vi "Thread 1.vi"(8 "error in (no error)":errorcluster, 11 "MyApp in":refnum<class "MyApp.lvclass">) -> (0 "error out":errorcluster, 3 "MyApp out":refnum<class "MyApp.lvclass">)   [LabVIEW 2012, in "MyApp.lvlib" / "MyApp.lvclass"]
uses:
  MyApp.lvclass
  HGF_LVC/HGF_BaseClasses/HGF_Event/HGF_Event.lvclass
  HGF_LVC/HGF_BaseClasses/HGF_Stop/HGF_Stop.lvclass
  HGF_LVC/HGF_BaseClasses/HGF_VariantDataObject/HGF_VariantDataObject.lvclass
  HGF_DataAnalyzer/WfmAnalysator/WfmAnalysator.lvclass
  HGF_DataAnalyzer/Wfm_Amplitude/Wfm_Amplitude.lvclass
  HGF_DataAnalyzer/Wfm_PulseMeasurement/Wfm_PulseMeasurement.lvclass
  MyApp.lvclass/MyApp.ctl
  HGF_DataAnalyzer/HGF_DataAnalysis/HGF_DataAnalysis.lvclass
  <vilib>/Utility/error.llb/DialogType.ctl
  <vilib>/measure/mascope.llb/Pulse Measurements 1 chan.vi
  <vilib>/measure/mascope.llb/Amplitude and Levels 1 chan.vi
  HGF_LVC/HGF_ApplicationBaseClasses/HGF_Application/HGF_Application.lvclass
  <vilib>/measure/NI_MABase.lvlib
  <vilib>/measure/NI_MAPro.lvlib
  HGF_LVC/HGF_BaseClasses/HGF_Composite/HGF_Composite.lvclass
panel:
  out "amplitude 3":dbl
  out "period 2":dbl format="%.2g"
  out "measurement info":T1
  out "Waveform Graph":waveform(dbl)(graph)
  out "low state level":dbl
  out "high state level":dbl
  out "amplitude 2":dbl format="%.2p"
  out "duty cycle":dbl
  out "pulse duration":dbl
  out "period":dbl format="%.2g"
  out "Analysis Error":errorcluster
  in  "sampling info":cluster{"Fs":dbl, "#s":dbl}={"Fs"=1000.0, "#s"=1000.0} {"Fs" format="%.2p"}
  in  "square wave duty cycle (%)":dbl=50.0 format="%0.2f"
  in  "amplitude":dbl=1.0 format="%0.2p"
  in  "frequency":dbl=10.0 format="%0.2p"
  in  "offset":dbl format="%0.2p"
  in  "signal type":T2(ring)
  in  "Generate Waveform":bool
  out "Iteration":i32
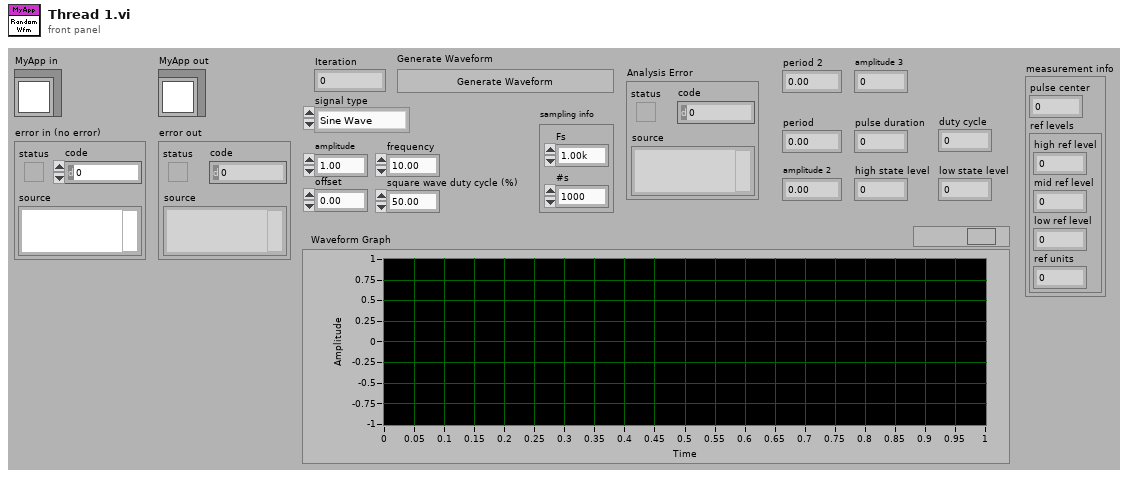
[diagram p1: front panel]
types:
  T1 = cluster{"pulse center":dbl, "ref levels":cluster{"high ref level":dbl, "mid ref level":dbl, "low ref level":dbl, "ref units":u16}}
  T2 = enum16{"Sine Wave", "Triangle Wave", "Square Wave", "Sawtooth Wave"}
  T3 = cluster{"seconds since 1Jan1904":timestamp, "message":string}
  T4 = typedef "DialogType.ctl" = u16
  T5 = cluster{"seconds since 1Jan1904":timestamp, string}
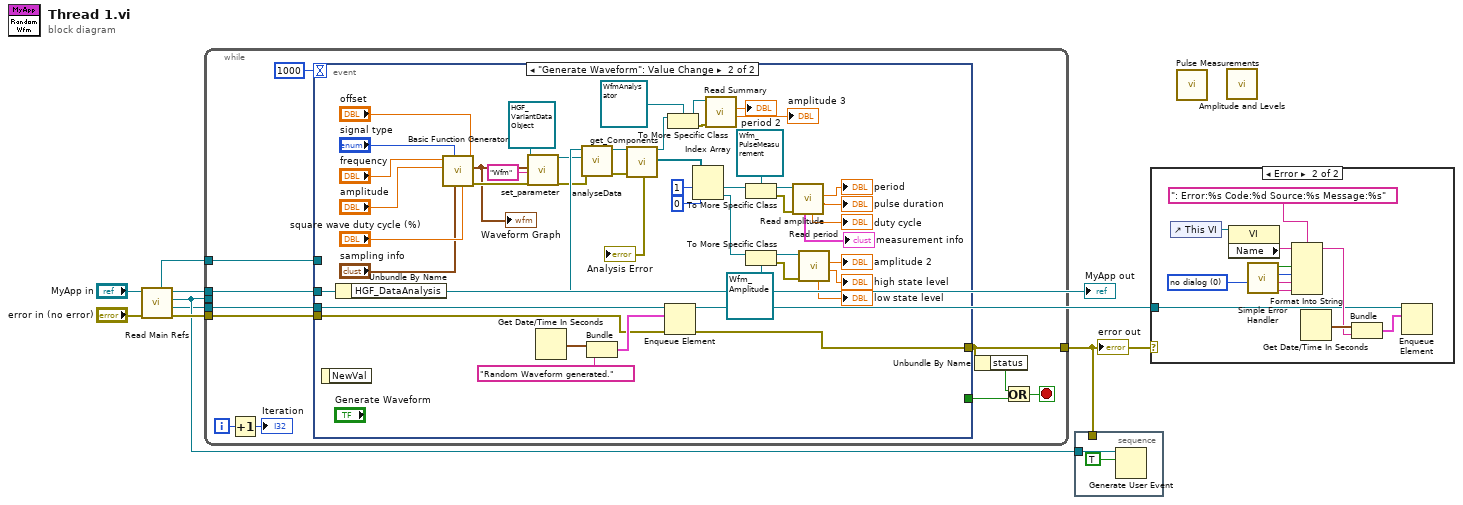
[diagram p0: block diagram]
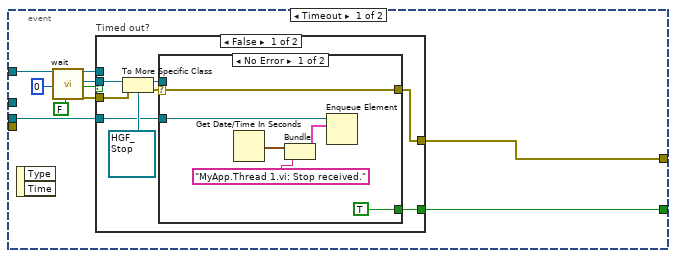
[diagram p3: hidden frame]
diagram:
  n1 = call "Read Main Refs.vi"("error in (no error)"="error in (no error)", "HGF_Application in"="MyApp in") -> ("error out"=w7:errorcluster, "Status Info Queue"=w3:refnum<queue>, "Main Stop Event"=w6:refnum<user-event>, "HGF_Application out"=w1:refnum<class "MyApp.lvclass">, "Info Event"=w8:refnum<class "HGF_Event.lvclass">)  [unwired: 2 in, 3 out]
  "MyApp out" <- w1
  n2 = while {
    tunnel: w6 -> [_]
    tunnel: w8 -> [w17]
    tunnel: w7 -> [w14]
    tunnel: w3 -> [w15]
    tunnel: [w12] -> w2
    tunnel: w1 -> [w9]
    i -> [w19]
    stop <- w11 stop-if-true
    n3 = Increment(x=w19) -> (x+1=→"Iteration":i32)
    n4 = event shown="[1] \"Generate Waveform\": Value Change" {
      selector: _ -> [_ _]
      dyn-events: _ -> [_ _]
      timeout: 1000 -> [_ _]
      tunnel: w17 -> [w25 _]
      tunnel: [w24 w88] -> w12
      tunnel: w15 -> [w21 w87]
      tunnel: w14 -> [_ w89]
      tunnel: [w22 _] -> w13
      tunnel: w9 -> [_ w77]
      event Timeout {
        n5 = event-data() -> ()  [unwired: 1 in, 2 out]
        n6 = call-dynamic "wait.vi"("HGF_Event"=w25, "msTimeout (-1)"=0, "ignore previous (F)"=FALSE) -> ("dup HGF_Event"=w28:refnum<class "HGF_Event.lvclass">, "Object"=w27:refnum<class>, "timed out"=w26:bool, "error out"=w29:errorcluster)  [unwired: 13 in]
        n7 = case "Timed out?" shown="False" w26 {
          tunnel: [w32 w45] -> w24
          tunnel: w29 -> [w36 w45]
          tunnel: w28 -> [_ _]
          tunnel: w27 -> [w37 _]
          tunnel: [w33 _] -> w22
          tunnel: w21 -> [w30 _]
          frame False {
            n8 = To More Specific Class(target class=refnum<class "HGF_Stop.lvclass"> refnum ("HGF_BaseClasses.lvlib:HGF_Stop.lvclass"), reference=w37, error in=w36) -> (specific class reference=w34:refnum<class "HGF_Stop.lvclass">, error out=w35:errorcluster)
            n9 = case shown="No Error" w35 {
              selector: w35 -> [w42 w44]
              tunnel: w34 -> [_ _]
              tunnel: [TRUE _] -> w33
              tunnel: [w42 w44] -> w32
              tunnel: w30 -> [w38 _]
              frame No Error {
                n10 = Get Date/Time In Seconds() -> (seconds since 1Jan1904=w40:timestamp)
                n11 = Bundle("seconds since 1Jan1904"=w40, "message"="MyApp.Thread 1.vi: Stop received.") -> (w41:T3)  [unwired: 1 in]
                n12 = Enqueue Element(queue=w38, element=w41) -> ()  [unwired: 2 in, 3 out]
              }
              frame Error {
              }
            }
          }
          frame True {
          }
        }
      }
      event "Generate Waveform": Value Change {
        n13 = event-data() -> ()  [unwired: 1 in, 1 out]
        n14 = Unbundle By Name(w77) -> ("HGF_DataAnalysis"=w76:refnum<class "HGF_DataAnalysis.lvclass">)
        n15 = call <vilib>:"Basic Function Generator.vi"("offset"="offset", "square wave duty cycle (%)"="square wave duty cycle (%)", "sampling info"="sampling info", "signal type"="signal type", "amplitude"="amplitude", "frequency"="frequency") -> ("error out"=w78:errorcluster, "signal out"=w66:waveform(dbl))  [unwired: 3 in, 1 out]
        "Waveform Graph" <- w66
        n16 = call "set_parameter.vi"("HGF_VariantDataObject"=refnum<class "HGF_VariantDataObject.lvclass"> refnum, "Parameter"=w66, "typeDescriptor"="Wfm", "error in (no error)"=w78) -> ("dup HGF_VariantDataObject"=w75:refnum<class "HGF_VariantDataObject.lvclass">, "error out"=w74:errorcluster)  [unwired: 14 in]
        n17 = Get Date/Time In Seconds() -> (seconds since 1Jan1904=w92:timestamp)
        n18 = call-dynamic "analyseData.vi"("error in (no error)"=w74, "HGF_VariantDataObject in"=w75, "HGF_DataAnalysis in"=w76) -> ("error out"=w72:errorcluster, "HGF_DataAnalysis out"=w73:refnum<class "HGF_DataAnalysis.lvclass">)  [unwired: 6 in, 1 out]
        n19 = Bundle("seconds since 1Jan1904"=w92, "message"="Random Waveform generated.") -> (w90:T3)  [unwired: 1 in]
        n20 = call "get_Components.vi"("HGF_Composite"=w73, "error in (no error)"=w72) -> ("dup HGF_Composite"=w62:refnum<class "HGF_DataAnalysis.lvclass">, "Components"=w63:refnum<class "HGF_Component.lvclass">[], "error out"=→"Analysis Error":errorcluster)  [unwired: 15 in]
        n21 = Enqueue Element(queue=w87, element=w90, error in (no error)=w89) -> (error out=w88:errorcluster)  [unwired: 1 in, 2 out]
        n22 = To More Specific Class(target class=refnum<class "WfmAnalysator.lvclass"> refnum ("MyApp.lvlib:WfmAnalysator.lvclass"), reference=w62) -> (specific class reference=w61:refnum<class "WfmAnalysator.lvclass">, error out=w65:errorcluster)  [unwired: 1 in]
        n23 = Index Array(array=w63, index #1=1 ("index"), index #2=0 ("index")) -> (element #1=w69:refnum<class "HGF_Component.lvclass">, element #2=w68:refnum<class "HGF_Component.lvclass">)
        n24 = call "Read Summary.vi"("error in (no error)"=w65, "WfmAnalysator in"=w61) -> ("amplitude"=→"amplitude 3":dbl, "period"=→"period 2":dbl)  [unwired: 6 in, 2 out]
        n25 = To More Specific Class(target class=refnum<class "Wfm_PulseMeasurement.lvclass"> refnum ("MyApp.lvlib:Wfm_PulseMeasurement.lvclass"), reference=w69) -> (specific class reference=w49:refnum<class "Wfm_PulseMeasurement.lvclass">, error out=w58:errorcluster)  [unwired: 1 in]
        n26 = To More Specific Class(target class=refnum<class "Wfm_Amplitude.lvclass"> refnum ("MyApp.lvlib:Wfm_Amplitude.lvclass"), reference=w68) -> (specific class reference=w47:refnum<class "Wfm_Amplitude.lvclass">, error out=w46:errorcluster)  [unwired: 1 in]
        n27 = call "Read amplitude.vi"("error in (no error)"=w58, "Wfm_PulseMeasurement in"=w49) -> ("pulse duration"=→"pulse duration":dbl, "period"=→"period":dbl, "duty cycle"=→"duty cycle":dbl, "measurement info"=→"measurement info":T1)  [unwired: 4 in, 2 out]
        n28 = call "Read period.vi"("error in (no error)"=w46, "Wfm_Amplitude in"=w47) -> ("high state level"=→"high state level":dbl, "amplitude"=→"amplitude 2":dbl, "low state level"=→"low state level":dbl)  [unwired: 5 in, 2 out]
      }
    }
    n29 = Unbundle By Name(w12) -> ("status"=w10:bool)
    n30 = Or(x=w10, y=w13) -> (x .or. y?=w11:bool)
  }
  "error out" <- w2
  n31 = stacked-sequence {
    tunnel: w6 -> [w94]
    tunnel: w2 -> [_]
    frame #0 {
      n32 = Generate User Event(user event=w94, event data cluster=TRUE ("event data")) -> ()  [unwired: 1 in, 2 out]
    }
  }
  n33 = case shown="Error" w2 {
    tunnel: w3 -> [_ w95]
    frame No Error {
    }
    frame Error {
      w97 = T4 0 items=["no dialog", "OK message", "continue or stop message", "OK message + warnings", "continue/stop + warnings"] ("type of dialog (OK msg:1)")
      n34 = control-ref of="This VI"() -> (w96:refnum<vi>)
      n35 = property class="VI"(reference=w96) -> ("Name"=w104:string)  [unwired: 1 in, 2 out]
      n36 = call <vilib>:"Simple Error Handler.vi"("type of dialog (OK msg:1)"=w97) -> ("error?"=w103:bool, "code out"=w102:i32, "source out"=w101:string, "message"=w100:string)  [unwired: 4 in, 1 out]
      n37 = Format Into String(format string=": Error:%s Code:%d Source:%s Message:%s", initial string=w104, w103, w102, w101, w100) -> (resulting string=w98:string)  [unwired: 1 in, 1 out]
      n38 = Get Date/Time In Seconds() -> (seconds since 1Jan1904=w106:timestamp)
      n39 = Bundle("seconds since 1Jan1904"=w106, w98) -> (w105:T5)  [unwired: 1 in]
      n40 = Enqueue Element(queue=w95, element=w105) -> ()  [unwired: 2 in, 3 out]
    }
  }
  n41 = call-poly <vilib>:"Pulse Measurements.vi"() -> ()  [unwired: 7 in, 5 out]
  n42 = call-poly <vilib>:"Amplitude and Levels.vi"() -> ()  [unwired: 8 in, 4 out]
